vi "Statistics Solver.vi"() -> ()   [LabVIEW 2023]
doc: "Determines the following statistics for each of the two input data sets: mean, median, mode, standard deviation, variance, skewness, RMS, and kurtosis. This example also computes combinational statistics between the two input data sets such as covariance, correlation, and MSE.\n\nNote: You must have the LabVIEW Full or Professional Development Systems to run this example."
uses:
  <vilib>/Analysis/baseanly.llb/Real A x B.vi
  <vilib>/Analysis/baseanly.llb/Complex A x B.vi
  <vilib>/Analysis/1siggen.llb/Ramp Pattern by Samples.vi
  <vilib>/Analysis/baseanly.llb/A x Vector.vi
  <vilib>/Analysis/7linalg.llb/Create Special Real Matrix.vi
  <vilib>/Analysis/7linalg.llb/Real Eigenvalues and Vectors.vi
  <vilib>/Analysis/7linalg.llb/Create Special Complex Matrix.vi
  <vilib>/Analysis/Matrix/Numeric/Complex/Complex To Cartesian - CM.vi
  <vilib>/Analysis/NI_AALPro.lvlib
  <vilib>/Analysis/NI_AALBase.lvlib
  <vilib>/gmath/NI_Gmath.lvlib
  <vilib>/Analysis/Matrix/NI_Matrix.lvlib
panel:
  out "correlation (Kendall)":dbl format="%#.6g"
  out "correlation (Spearman)":dbl format="%#.6g"
  out "mean of y":dbl format="%#.6g"
  out "variance of y":dbl format="%#.6g"
  out "Histogram x":T1(graph)
  out "Time Chart Y":cluster{dbl[], dbl[]}(graph)
  out "Time Chart X":cluster{dbl[], dbl[]}(graph)
  out "variance of x":dbl format="%#.6g"
  out "mean of x":dbl format="%#.6g"
  out "mean square error (MSE)":dbl format="%#.6g"
  out "correlation (r)":dbl format="%#.6g"
  in  "Correlation of X and Y":dbl(slide)=0.7 scale=-1.0..1.0
  in  "Variance of y":dbl=1.5
  in  "Variance of x":dbl=2.0
  in  "Average y":dbl(slide) scale=-10.0..10.0
  in  "Average x":dbl(slide) scale=-10.0..10.0
  in  "Seed":i32=-1
  out "Scatter Plot":cluster{dbl[], dbl[]}[](graph)
  out "Histogram Y":T2(graph)
  in  "Stop":bool
  out "Covariance of x and y":dbl format="%#.6g"
  # "Overview: Determines statistics for each of the two input data sets.\nRequirements: LabVIEW Full Development System\nInstructions: \n1. Run the VI.\n2. Change parameters of signal x and y and see how this affects the correlation parameters.\n3. Modify the Correlation of X and Y and see the data skewed to one direction.\n4. Click Stop to stop the VI."
  # "Measured Statistical Parameters"
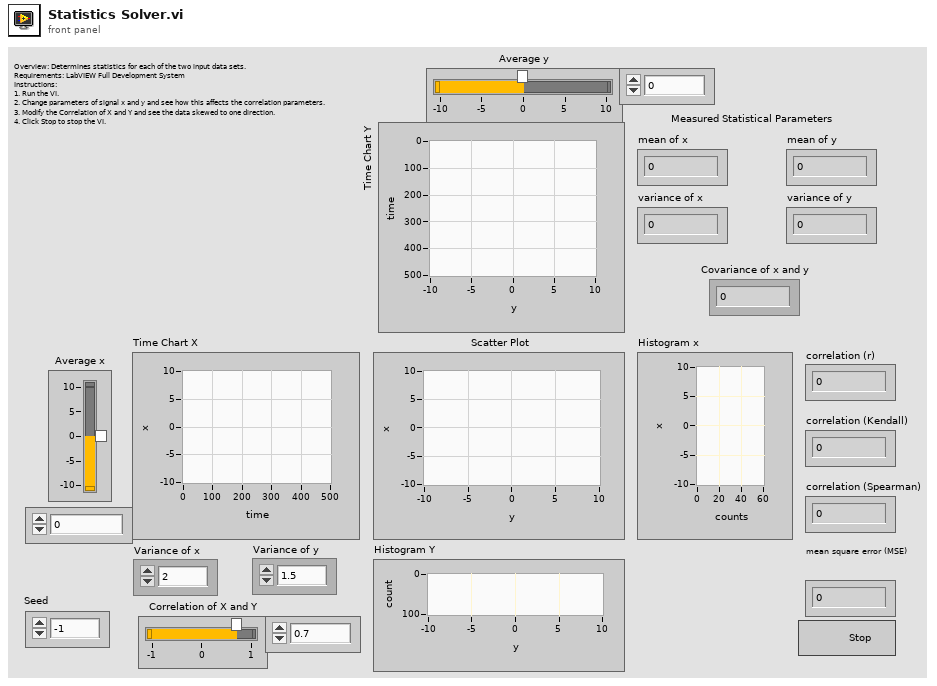
[diagram p1: front panel]
types:
  T1 = cluster{"Histogram: h(x)":i32[], "X Values":dbl[]}
  T2 = cluster{"X Values":dbl[], "Histogram: h(x)":i32[]}
  T3 = typedef "NI_Matrix.lvlib/RealMatrix.ctl" = dbl[][]
  T4 = typedef "NI_Matrix.lvlib/ComplexMatrix.ctl" = cdb[][]
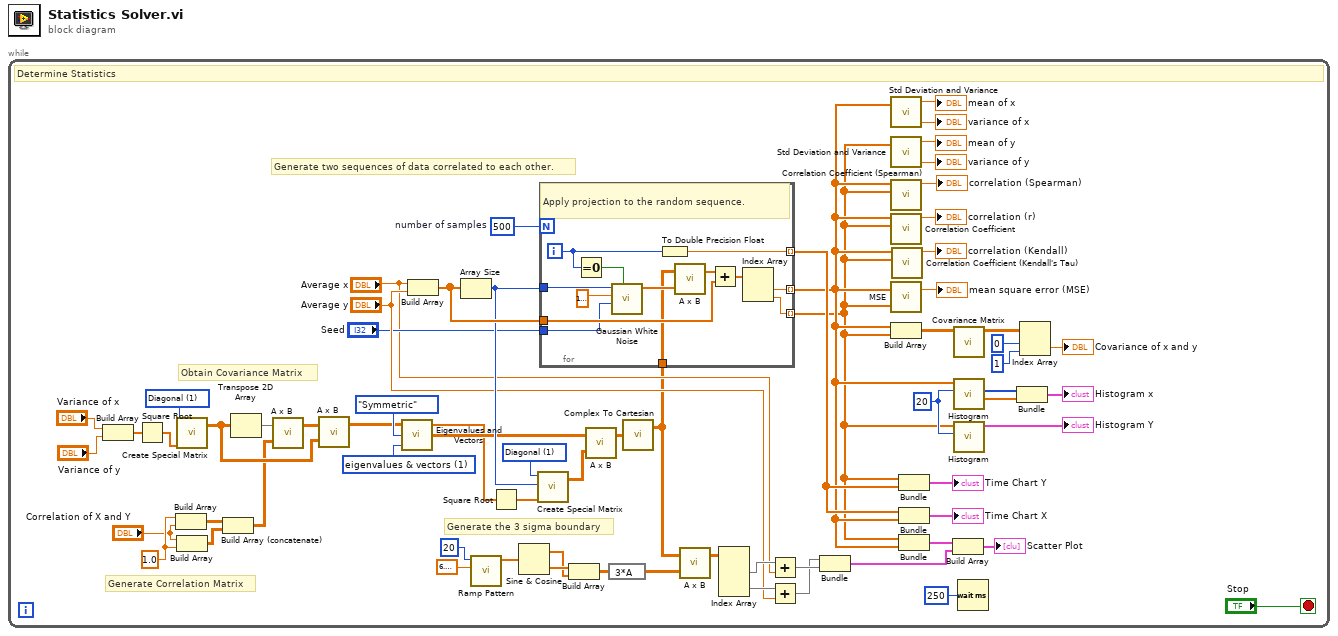
[diagram p0: block diagram]
diagram:
  n1 = while {
    stop <- "Stop" stop-if-true
    w1 = 1 items=["Identity", "Diagonal", "Toeplitz", "Vandermonde", "Companion", "Hankel", "Hadamard", "Wilkinson", "Hilbert", "Inverse Hilbert", "Rosser", "Pascal"] ("matrix type")
    w20 = 1.0
    w24 = 1 items=["Identity", "Diagonal", "Toeplitz", "Vandermonde", "Companion", "Hankel", "Hadamard", "Wilkinson", "Hilbert", "Inverse Hilbert", "Rosser", "Pascal"] ("matrix type")
    w69 = 20 ("intervals")
    w56 = 1 items=["eigenvalues", "eigenvalues & vectors"] ("output option")
    w41 = 500  # number of samples
    # "Generate the 3 sigma boundary"
    # "Generate two sequences of data correlated to each other."
    # "Obtain Covariance Matrix"
    # "Generate Correlation Matrix"
    # "Determine Statistics"
    n2 = Build Array("Variance of x", "Variance of y") -> (w18:dbl[])
    n3 = Square Root(x=w18) -> (sqrt(x)=w12:dbl[])
    n4 = Build Array(w20, "Correlation of X and Y") -> (w54:T3)
    n5 = call-poly <vilib>:"Create Special Matrix.vi"("matrix type"=w24, "Input Vector1"=w12) -> ("Special Matrix"=w22:T3)  [unwired: 3 in, 1 out]
    n6 = Build Array("Correlation of X and Y", w20) -> (w53:T3)
    n7 = Build Array (concatenate)(w54, w53) -> (w17:T3)
    n8 = Transpose 2D Array(2D array=w22) -> (transposed array=w23:T3)
    n9 = call-poly <vilib>:"A x B.vi"("B"=w17, "A"=w23) -> ("A x B"=w21:T3)  [unwired: 1 out]
    n10 = call-poly <vilib>:"A x B.vi"("B"=w22, "A"=w21) -> ("A x B"=w16:T3)  [unwired: 1 out]
    n11 = call-poly <vilib>:"Eigenvalues and Vectors.vi"("output option"=w56, "matrix type"=enum32{"General", "Symmetric"}."Symmetric", "Input Matrix"=w16) -> ("Eigenvectors"=w59:T4, "Eigenvalues"=w52:cdb[])  [unwired: 1 out]
    n12 = Build Array("Average x", "Average y") -> (w61:dbl[])
    n13 = Array Size(array=w61) -> (size(s)=w60:i32)
    n14 = call-poly <vilib>:"Ramp Pattern.vi"("end"=6.283185307179586, "samples"=20) -> ("Ramp Pattern"=w43:dbl[])  [unwired: 8 in, 1 out]
    n15 = Square Root(x=w52) -> (sqrt(x)=w58:cdb[])
    n16 = Sine & Cosine(0:w43) -> (1:w42:dbl[], 2:w62:dbl[])
    n17 = call-poly <vilib>:"Create Special Matrix.vi"("matrix type"=w1, "matrix size"=w60, "Input Vector1"=w58) -> ("Special Matrix"=w57:T4)  [unwired: 1 in, 2 out]
    n18 = Build Array(w62, w42) -> (w10:dbl[][])
    n19 = call-poly <vilib>:"A x B.vi"("B"=w57, "A"=w59) -> ("A x B"=w51:T4)  [unwired: 1 out]
    n20 = expression code="3*A"(w10) -> (w9:dbl[][])
    n21 = call-poly <vilib>:"Complex To Cartesian.vi"("Complex Matrix R + Ii"=w51) -> ("Real Matrix R"=w8:T3)  [unwired: 1 out]
    n22 = for {
      N: w41 -> [_]
      tunnel: [w82] -> w6 mode=indexing
      tunnel: [w81] -> w7 mode=indexing
      tunnel: w61 -> [w80]
      tunnel: w60 -> [w78]
      tunnel: w8 -> [w73]
      tunnel: [w70] -> w38 mode=indexing
      tunnel: "Seed" -> [w71]
      i -> [w72]
      # "Apply projection to the random sequence."
      n23 = Equal To 0?(x=w72) -> (x = 0?=w75:bool)
      n24 = call <vilib>:"Gaussian White Noise.vi"("initialize?"=w75, "seed"=w71, "standard deviation"=1.0000000000000002, "samples"=w78) -> ("Gaussian noise pattern"=w74:dbl[])  [unwired: 6 in, 1 out]
      n25 = To Double Precision Float(number=w72) -> (double precision float=w70:dbl)
      n26 = call-poly <vilib>:"A x B.vi"("Vector"=w74, "A"=w73) -> ("A x Vector"=w76:dbl[])  [unwired: 1 out]
      n27 = Add(x=w76, y=w80) -> (x+y=w79:dbl[])
      n28 = Index Array(array=w79) -> (element #1=w81:dbl, element #2=w82:dbl)  [unwired: 2 in]
    }
    n29 = call-poly <vilib>:"A x B.vi"("B"=w9, "A"=w8) -> ("A x B"=w48:T3)  [unwired: 1 out]
    n30 = Index Array(array=w48) -> (element #1=w50:dbl[], element #2=w49:dbl[])  [unwired: 4 in]
    n31 = Add(x=w50, y="Average x") -> (x+y=w32:dbl[])
    n32 = Add(x=w49, y="Average y") -> (x+y=w31:dbl[])
    n33 = Bundle(w31, w32) -> (w44:cluster{dbl[], dbl[]})  [unwired: 1 in]
    n34 = call <vilib>:"Std Deviation and Variance.vi"("X"=w7) -> ("mean"=→"mean of x":dbl, "variance"=→"variance of x":dbl)  [unwired: 1 in, 1 out]
    n35 = call <vilib>:"Std Deviation and Variance.vi"("X"=w6) -> ("mean"=→"mean of y":dbl, "variance"=→"variance of y":dbl)  [unwired: 1 in, 1 out]
    n36 = call <vilib>:"Correlation Coefficient (Spearman).vi"("Y"=w6, "X"=w7) -> ("correlation coefficient r"=→"correlation (Spearman)":dbl)  [unwired: 8 in, 1 out]
    n37 = call <vilib>:"Correlation Coefficient.vi"("Y"=w6, "X"=w7) -> ("correlation coefficient r"=→"correlation (r)":dbl)  [unwired: 8 in, 1 out]
    n38 = call <vilib>:"MSE.vi"("X Values"=w6, "Y Values"=w7) -> ("mse"=→"mean square error (MSE)":dbl)  [unwired: 1 out]
    n39 = Build Array(w7, w6) -> (w29:T3)
    n40 = call <vilib>:"Correlation Coefficient (Kendall's Tau).vi"("Y"=w6, "X"=w7) -> ("correlation coefficient r"=→"correlation (Kendall)":dbl)  [unwired: 8 in, 1 out]
    n41 = Bundle(w6, w38) -> (→"Time Chart Y":cluster{dbl[], dbl[]})  [unwired: 1 in]
    n42 = Bundle(w38, w7) -> (→"Time Chart X":cluster{dbl[], dbl[]})  [unwired: 1 in]
    n43 = Bundle(w6, w7) -> (w46:cluster{dbl[], dbl[]})  [unwired: 1 in]
    n44 = Build Array(w46, w44) -> (→"Scatter Plot":cluster{dbl[], dbl[]}[])
    n45 = call <vilib>:"Covariance Matrix.vi"("X"=w29) -> ("covariance matrix V"=w30:T3)  [unwired: 9 in, 1 out]
    n46 = call <vilib>:"Histogram.vi"("intervals"=w69, "X"=w7) -> ("X Values"=w35:dbl[], "Histogram: h(x)"=w36:i32[])  [unwired: 6 in, 2 out]
    n47 = call <vilib>:"Histogram.vi"("intervals"=w69, "X"=w6) -> ("Histogram Graph"=→"Histogram Y":T2)  [unwired: 6 in, 3 out]
    n48 = Wait (ms)(milliseconds to wait=u32 250 ("millisecond multiple")) -> ()  [unwired: 1 out]
    n49 = Bundle("Histogram: h(x)"=w36, "X Values"=w35) -> (→"Histogram x":T1)  [unwired: 1 in]
    n50 = Index Array(array=w30, index (row)=0, index (col)=1) -> (element=→"Covariance of x and y":dbl)
  }
